vi "Element Init.vi"(7 "VolatusAPI":refnum<class "VolatusAPI.lvclass">, 8 "error in (no error)":errorcluster, 10 "JSON":string, 11 "ImageButtonControl in":refnum<class "ImageButtonControl.lvclass">) -> (0 "error out":errorcluster, 3 "ImageButtonControl out":refnum<class "ImageButtonControl.lvclass">)   [LabVIEW 2020, in "VolatusGUIElements.lvlib" / "ImageButtonControl.lvclass"]
uses:
  ImageButtonControl.lvclass
  C:/dev/lv20CE/relink/lv-volatus/VolatusGUI/GUI Element/GUI Element.lvclass
  Volatus/VolatusAPI/VolatusAPI.lvclass
  lv-vecto/Vecto/Group DBL/Group DBL.lvclass
  C:/dev/lv20CE/relink/lv-vecto/Vecto/Group/Group.lvclass
  JSON.ctl
  VolatusGUI/GUI Element/GUI Element.lvclass/GUI Element.ctl
  ImageButtonControl.lvclass/ImageButtonControl.ctl
  353c6030-d962-46c0-a067-67411140a0fa.vi
  <vilib>/JDP Science/JSONtext/JSON text to Variant.vi
  <vilib>/JDP Science/JSONtext/LVClass Serializer/JSONtext LVClass Serializer.lvclass
  VolatusGUI/GUI Element/GUI Element.lvclass
  volatus-gui-controls/VolatusGUIEditorCore/VolatusGUIEditorCore.lvlib
  VolatusGUI/Element Inhibit/Element Inhibit.lvclass
  Volatus/Digital Command/Digital Command.lvclass
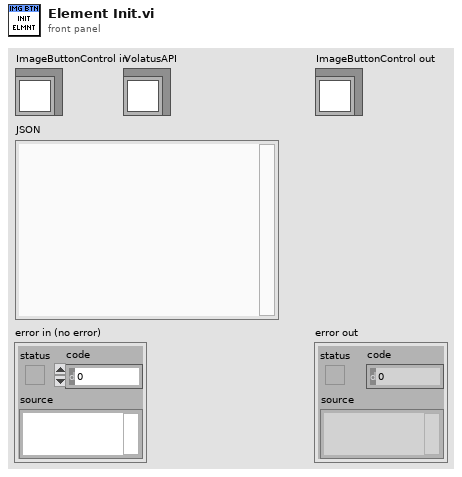
[diagram p1: front panel]
types:
  T1 = typedef "VolatusGUIElements.lvlib/ImageButtonControl.lvclass/JSON.ctl" = cluster{"Channel":string, "FalseImage":string, "TrueImage":string, "Inhibit":string}
  T2 = typedef "VectoConfig.lvlib/Channel Info.ctl" = cluster{"Name":string, "Group":string, "Owning Node":string, "Owning Task":string, "Resource":string}
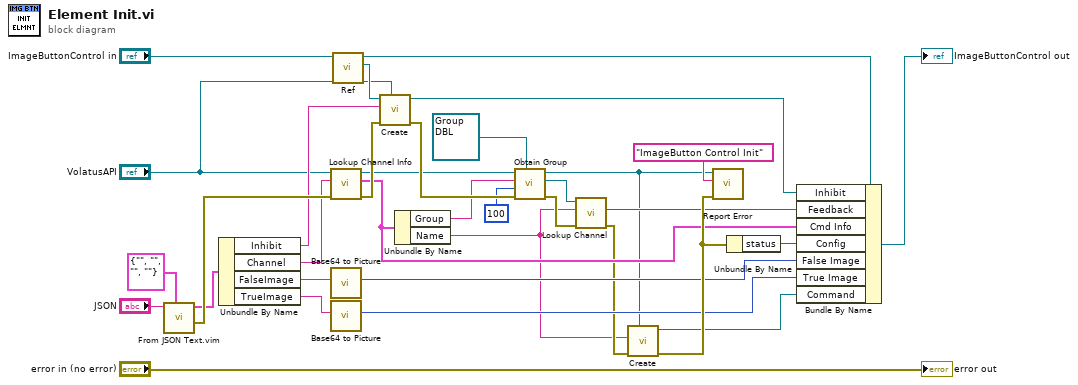
[diagram p0: block diagram]
diagram:
  n1 = call "From JSON Text.vim"("Data Type and Default Value"=T1 {"Channel"="", "FalseImage"="", "TrueImage"="", "Inhibit"=""} ("JSON"), "JSON"="JSON") -> ("error out"=w31:errorcluster, "Data out"=w25:T1)  [unwired: 8 in]
  n2 = Unbundle By Name(w25) -> ("Inhibit"=w8:string, "Channel"=w23:string, "FalseImage"=w13:string, "TrueImage"=w12:string)
  n3 = call "Lookup Channel Info.vi"("error in (no error)"=w31, "Channel Name"=w23, "VolatusAPI in"="VolatusAPI") -> ("error out"=w32:errorcluster, "Channel Info"=w20:T2, "VolatusAPI out"=w24:refnum<class "VolatusAPI.lvclass">)  [unwired: 5 in, 1 out]
  n4 = call "Base64 to Picture.vi"("Base64 PNG Data"=w13) -> ("Picture"=w11:picture)  [unwired: 9 in, 1 out]
  n5 = call "Base64 to Picture.vi"("Base64 PNG Data"=w12) -> ("Picture"=w10:picture)  [unwired: 9 in, 1 out]
  n6 = call "Ref.vi"("GUI Element in"="ImageButtonControl in") -> ("Ref"=w9:refnum<vi>, "GUI Element out"=w30:refnum<class "ImageButtonControl.lvclass">)  [unwired: 9 in]
  n7 = call "Create.vi"("VolatusAPI"="VolatusAPI", "error in (no error)"=w32, "Inhibit Channel"=w8, "Control Ref"=w9) -> ("error out"=w33:errorcluster, "Element Inhibit out"=w6:refnum<class "Element Inhibit.lvclass">)  [unwired: 6 in]
  n8 = Unbundle By Name(w20) -> ("Group"=w21:string, "Name"=w3:string)
  n9 = call "Obtain Group.vi"("Group Type (Abstract)"=refnum<class "Group DBL.lvclass"> refnum ("Vecto.lvlib:Group.lvclass"), "error in (no error)"=w33, "Timeout ms (5000)"=u32 100, "Group Name"=w21, "VolatusAPI in"=w24) -> ("error out"=w27:errorcluster, "Group"=w28:refnum<class "Group DBL.lvclass">, "VolatusAPI out"=w2:refnum<class "VolatusAPI.lvclass">)  [unwired: 4 in]
  n10 = call "Lookup Channel.vi"("error in (no error)"=w27, "Channel Name"=w3, "Group in"=w28) -> ("error out"=w4:errorcluster, "Channel"=w26:refnum<class "Channel DBL.lvclass">)  [unwired: 6 in, 1 out]
  n11 = call "Create.vi"("VolatusAPI"=w2, "error in (no error)"=w4, "Channel"=w3) -> ("error out"=w34:errorcluster, "Digital Command out"=w5:refnum<class "Digital Command.lvclass">)  [unwired: 7 in]
  n12 = call "Report Error.vi"("error in (no error)"=w34, "Context"="ImageButton Control Init", "VolatusAPI in"=w2) -> ()  [unwired: 7 in, 2 out]
  n13 = Unbundle By Name(w34) -> ("status"=w22:bool)
  n14 = Bundle By Name(cluster=w30, "Inhibit"=w6, "Feedback"=w26, "Cmd Info"=w20, "Config"=w22, "False Image"=w11, "True Image"=w10, "Command"=w5) -> (→"ImageButtonControl out":refnum<class "ImageButtonControl.lvclass">)
  "error out" <- "error in (no error)"
